vi "Capture.vi"(0 "Commands array":string[][](array[string])=[["Group20.825", "Group20.671", "Group20.814", "Group30.121"], ["Group2-0.528", "Group2-1.243", "Group2-0.539", "Group30.121"], ["Group20.374", "Group21.573", "Group20.363", "Group30.121"], ["Group2-0.242", "Group2-1.815", "Group2-0.253", "Group30.121"], ["Group20.165", "Group21.991", "Group20.154", "Group30.121"], ["Group2-0.077", "Group2-2.145", "Group2-0.088", "Group30.121"], ["Group20.044", "Group22.233", "Group20.033", "Group30.121"], ["Group2-2.310", "WT10", "WT10", "Group30.121"], ["Group22.310", "WT10", "WT10", "Group30.121"], ["Group2-2.310", "WT10", "WT10", "Group30.121"], ["Group22.310", "WT10", "WT10", "Group30.121"], ["Group2-2.310", "WT10", "WT10", "Group30.121"], ["Group22.310", "WT10", "WT10", "Group30.121"], ["Group2-0.011", "Group2-2.277", "Group2-0.022", "Group30.121"], ["Group20.066", "Group22.189", "Group20.055", "Group30.121"], ["Group2-0.121", "Group2-2.057", "Group2-0.132", "Group30.121"], ["Group20.209", "Group21.903", "Group20.198", "Group30.121"], ["Group2-0.297", "Group2-1.705", "Group2-0.308", "Group30.121"], ["Group20.451", "Group21.419", "Group20.440", "Group30.121"], ["Group2-0.660", "Group2-0.979", "Group2-0.671", "Group30.121"]], 1 "XPS_Address":string="192.168.254.254", 2 "VISA resource name":refnum<visa-resource-name>, 3 "laser array index":i32, 4 "Process time":dbl format="%#_13g", 5 "Axis Speed":dbl=1.0 format="%#_13g", 6 "Laser on/off array":bool[][](array[boolean])=[[FALSE, TRUE, FALSE, FALSE], [FALSE, TRUE, FALSE, FALSE], [FALSE, TRUE, FALSE, FALSE], [FALSE, TRUE, FALSE, FALSE], [FALSE, TRUE, FALSE, FALSE], [FALSE, TRUE, FALSE, FALSE], [FALSE, TRUE, FALSE, FALSE], [TRUE, FALSE, FALSE, FALSE], [TRUE, FALSE, FALSE, FALSE], [TRUE, FALSE, FALSE, FALSE], [TRUE, FALSE, FALSE, FALSE], [TRUE, FALSE, FALSE, FALSE], [TRUE, FALSE, FALSE, FALSE], [FALSE, TRUE, FALSE, FALSE], [FALSE, TRUE, FALSE, FALSE], [FALSE, TRUE, FALSE, FALSE], [FALSE, TRUE, FALSE, FALSE], [FALSE, TRUE, FALSE, FALSE], [FALSE, TRUE, FALSE, FALSE], [FALSE, TRUE, FALSE, FALSE]], 7 "stop":bool, 8 "delay before read (ms)":u32=500, 11 "Axis Initial Parameters":T1={"Velocity (units/seconds)"=1.0, "Acceleration (units/seconds²)"=20.0, "Minimum Jerk Time (seconds)"=0.005, "Maximum Jerk Time (seconds)"=0.009} {"Maximum Jerk Time (seconds)" format="%.6e"; "Minimum Jerk Time (seconds)" format="%.6e"; "Acceleration (units/seconds²)" format="%.6e"; "Velocity (units/seconds)" format="%.6e"}, 13 "ROI Area \n(mm2)":dbl=4.035870075999999, 14 "Axis 2":string="Group3", 15 "Axis 1":string="Group2", 17 "OPO on?":bool, 19 "Acceleration (units/seconds²)":dbl=20.0) -> (10 "Elapsed time":dbl, 16 "XPS error out":errorcluster, 18 "Error out":errorcluster)   [LabVIEW 2016]
uses:
  case selector.ctl
panel:
  out "Capture Log":string
  out "Axis 1 position":dbl format="%.10f"
  out "Axis 2 position":dbl format="%.10f"
  out "Initial time":timestamp
  in  "Active Positioner":string
  out "Current Line":i32
  out "1D Laser Array":bool[](array[boolean])=[FALSE, TRUE, FALSE, FALSE, FALSE, TRUE, FALSE, FALSE, FALSE, TRUE, FALSE, FALSE, FALSE, TRUE, FALSE, FALSE, FALSE, TRUE, FALSE, FALSE, FALSE, TRUE, FALSE, FALSE, FALSE, TRUE, FALSE, FALSE, TRUE, FALSE, FALSE, FALSE, TRUE, FALSE, FALSE, FALSE, TRUE, FALSE, FALSE, FALSE, TRUE, FALSE, FALSE, FALSE, TRUE, FALSE, FALSE, FALSE, TRUE, FALSE, FALSE, FALSE, FALSE, TRUE, FALSE, FALSE, FALSE, TRUE, FALSE, FALSE, FALSE, TRUE, FALSE, FALSE, FALSE, TRUE, FALSE, FALSE, FALSE, TRUE, FALSE, FALSE, FALSE, TRUE, FALSE, FALSE, FALSE, TRUE, FALSE, FALSE]
  out "1D command array":string[](array[string])=["Group20.825", "Group20.671", "Group20.814", "Group30.121", "Group2-0.528", "Group2-1.243", "Group2-0.539", "Group30.121", "Group20.374", "Group21.573", "Group20.363", "Group30.121", "Group2-0.242", "Group2-1.815", "Group2-0.253", "Group30.121", "Group20.165", "Group21.991", "Group20.154", "Group30.121", "Group2-0.077", "Group2-2.145", "Group2-0.088", "Group30.121", "Group20.044", "Group22.233", "Group20.033", "Group30.121", "Group2-2.310", "WT10", "WT10", "Group30.121", "Group22.310", "WT10", "WT10", "Group30.121", "Group2-2.310", "WT10", "WT10", "Group30.121", "Group22.310", "WT10", "WT10", "Group30.121", "Group2-2.310", "WT10", "WT10", "Group30.121", "Group22.310", "WT10", "WT10", "Group30.121", "Group2-0.011", "Group2-2.277", "Group2-0.022", "Group30.121", "Group20.066", "Group22.189", "Group20.055", "Group30.121", "Group2-0.121", "Group2-2.057", "Group2-0.132", "Group30.121", "Group20.209", "Group21.903", "Group20.198", "Group30.121", "Group2-0.297", "Group2-1.705", "Group2-0.308", "Group30.121", "Group20.451", "Group21.419", "Group20.440", "Group30.121", "Group2-0.660", "Group2-0.979", "Group2-0.671", "Group30.121"]
  out "Current Command":string
  out "Current laser element":bool
  out "Total lines":i32=80
  in  "Active Axis":string
  out "Laser on/off":bool
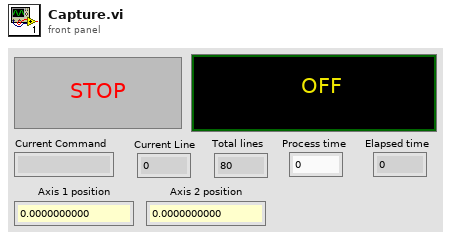
[diagram p1: front panel]
types:
  T1 = cluster{"Velocity (units/seconds)":dbl, "Acceleration (units/seconds²)":dbl, "Minimum Jerk Time (seconds)":dbl, "Maximum Jerk Time (seconds)":dbl}
  T2 = typedef "case selector.ctl" = enum16{"Initialize", "Element selection", "Laser", "Velocities", "Command", "Wait", "Exit"}
  T3 = enum16{"open", "replace", "create", "open or create", "replace or create", "replace or create with confirmation"}
  T4 = cluster{"connection TCP":refnum<k5>, "LogTo File":bool, "Log File refnum":refnum<file>, "no error if error log":bool}
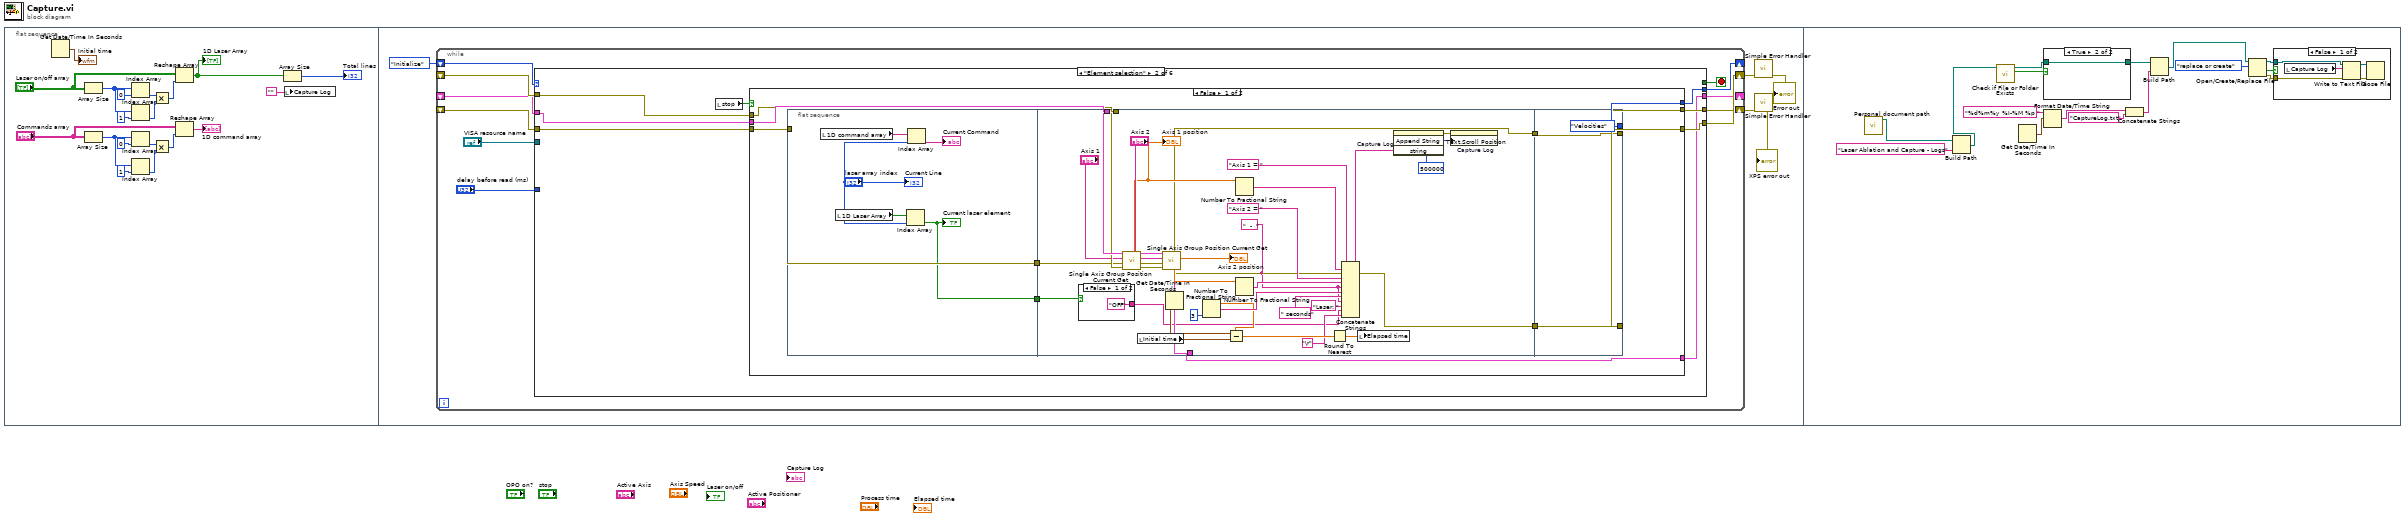
[diagram p0: block diagram]
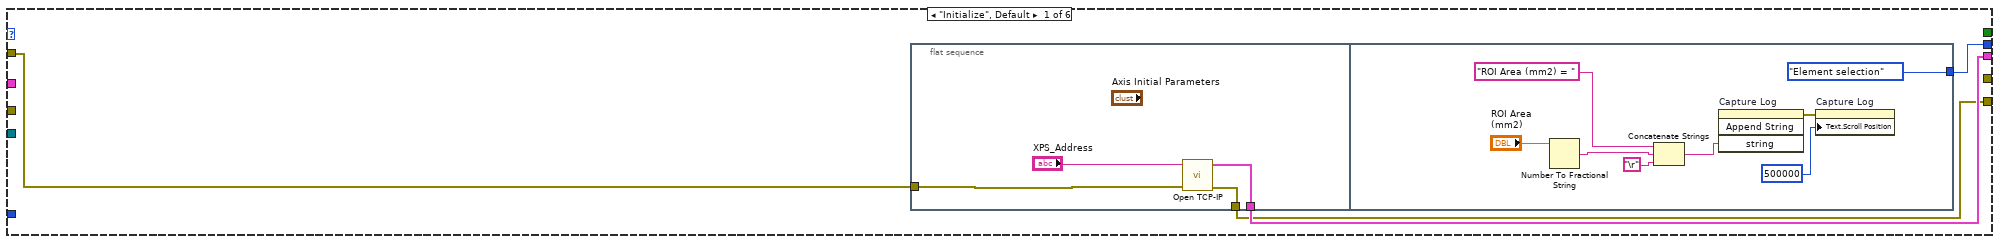
[diagram p2: hidden frame]
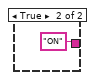
[diagram p3: hidden frame]
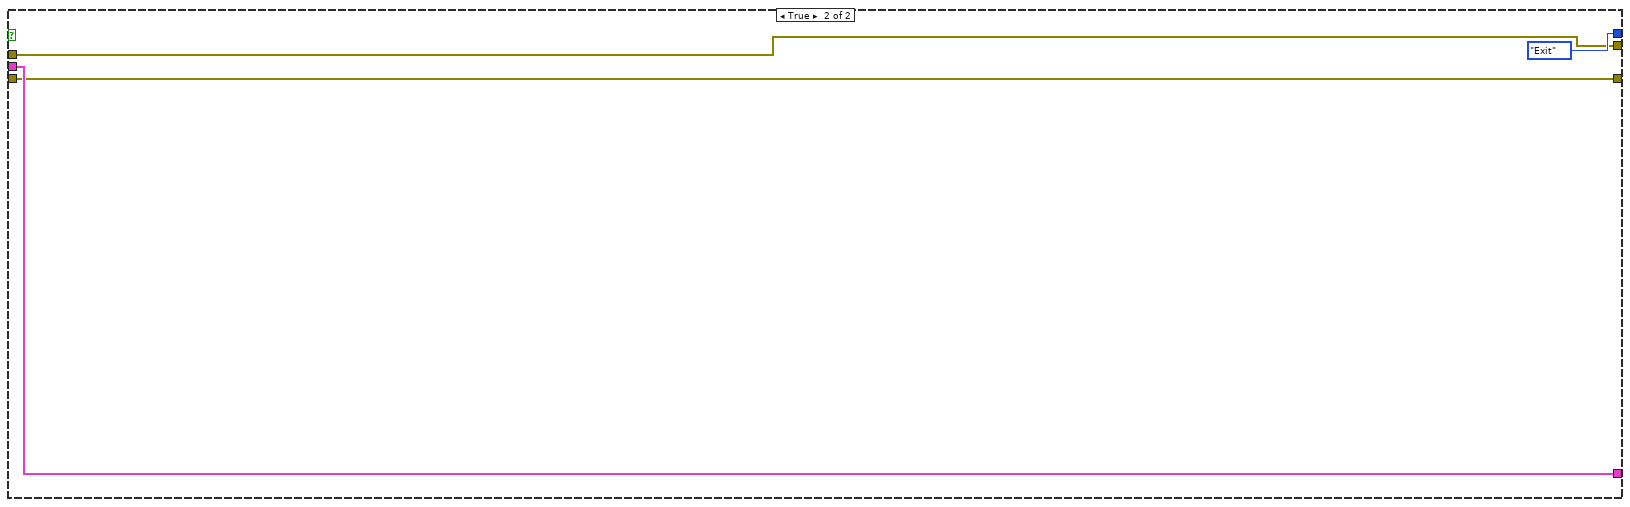
[diagram p4: hidden frame]
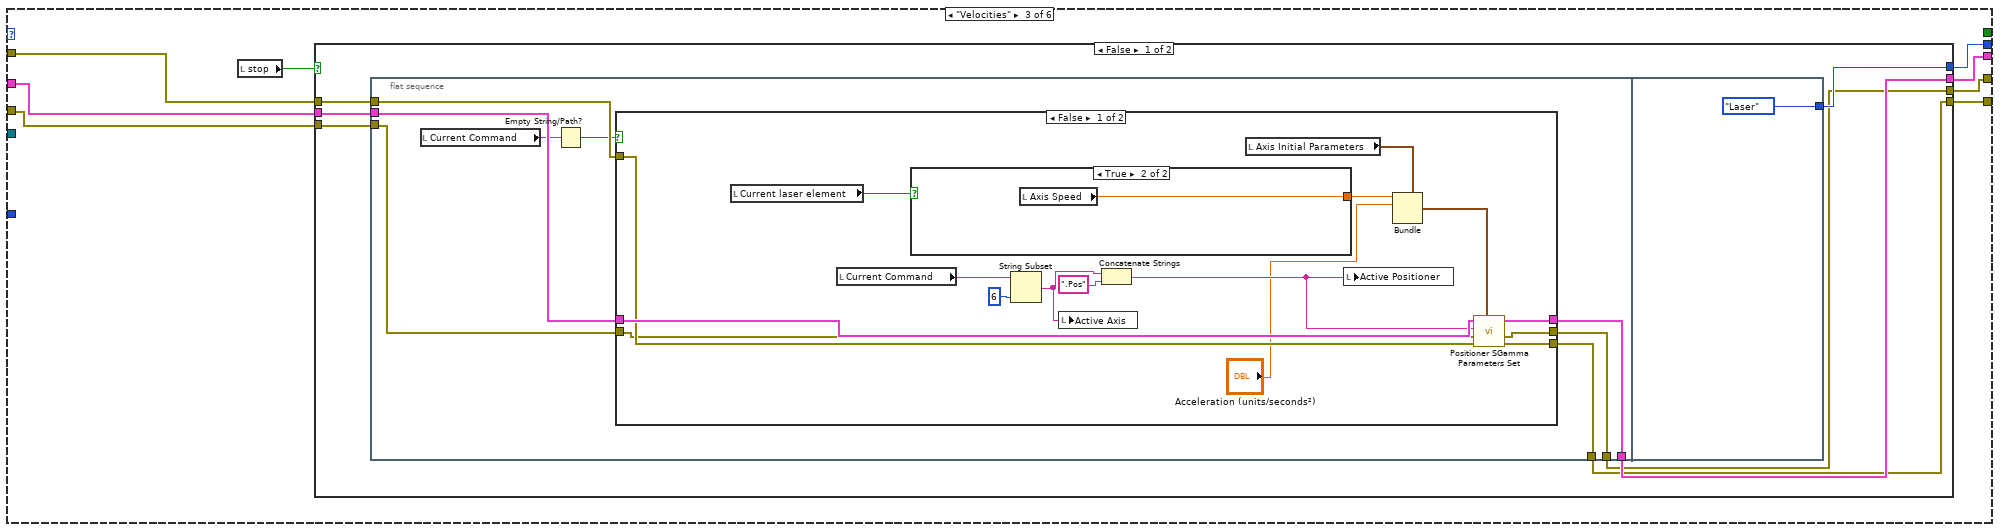
[diagram p5: hidden frame]
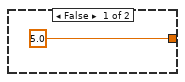
[diagram p6: hidden frame]
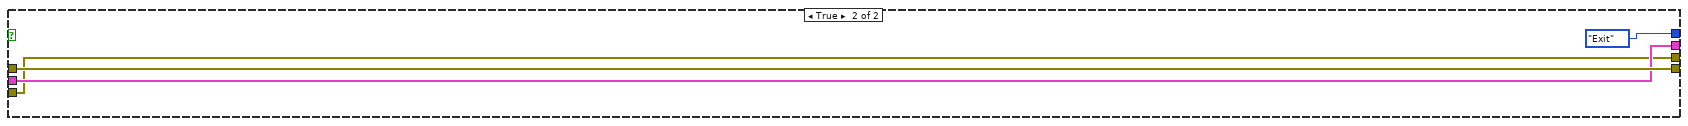
[diagram p8: hidden frame]
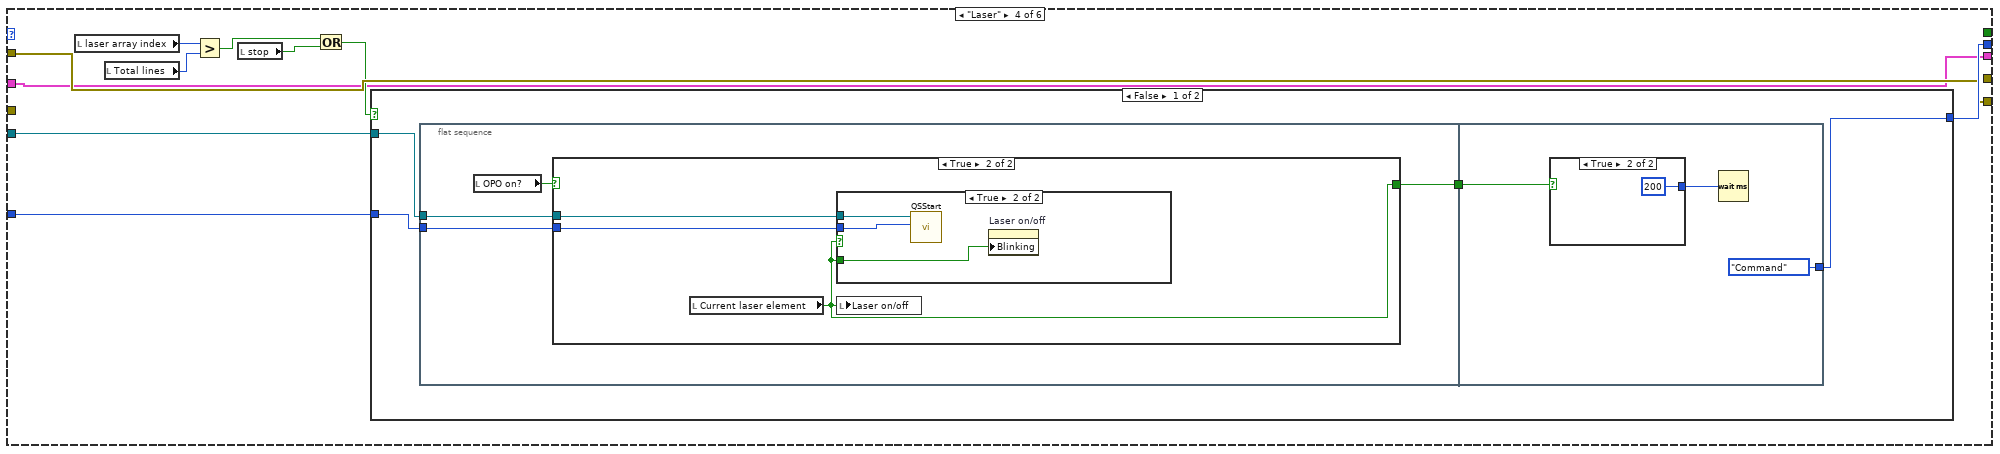
[diagram p9: hidden frame]
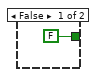
[diagram p10: hidden frame]
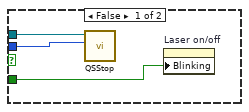
[diagram p11: hidden frame]
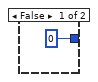
[diagram p12: hidden frame]
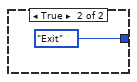
[diagram p13: hidden frame]
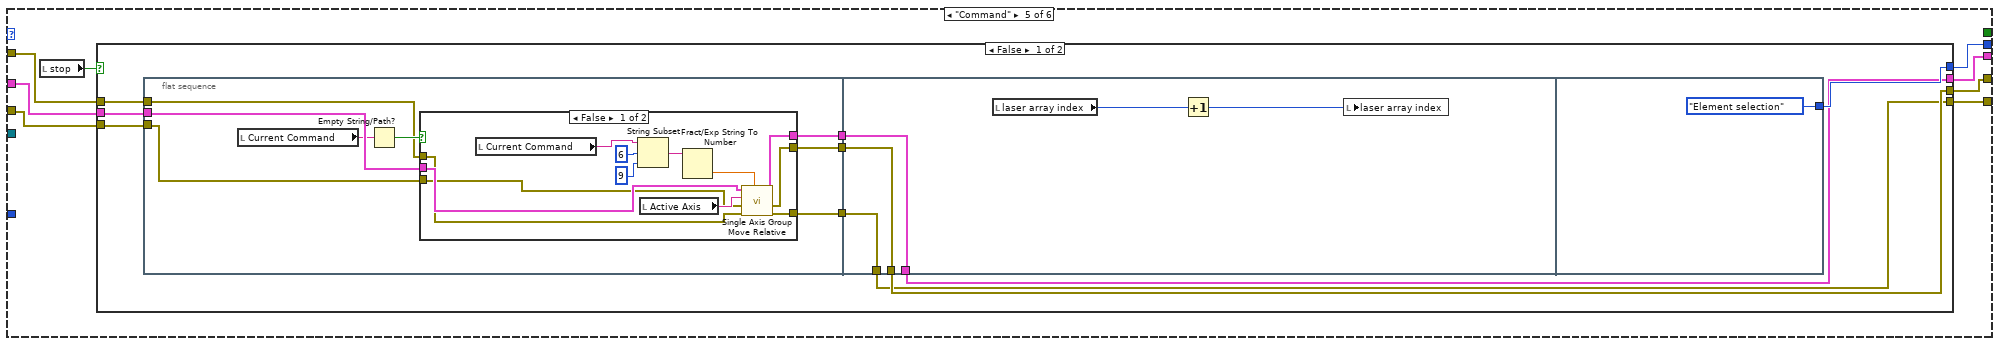
[diagram p14: hidden frame]
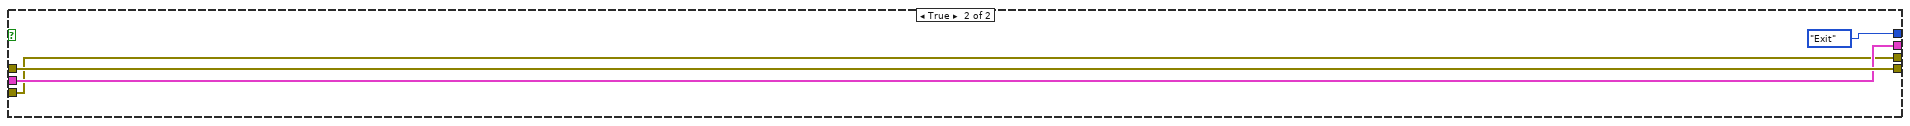
[diagram p16: hidden frame]
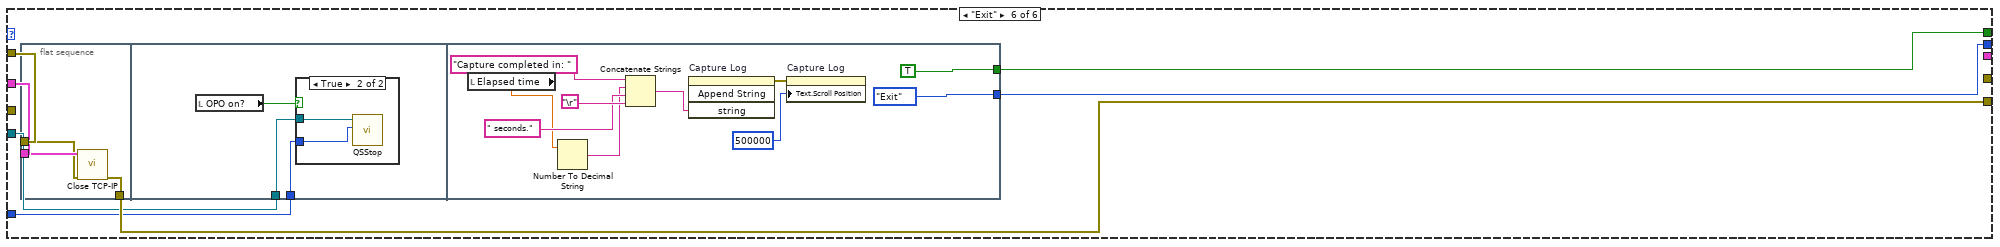
[diagram p17: hidden frame]
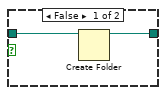
[diagram p19: hidden frame]
diagram:
  n1 = flat-sequence {
    frame #0 {
      n2 = Get Date/Time In Seconds() -> (seconds since 1Jan1904=→"Initial time":timestamp)
      n3 = Array Size(array="Commands array") -> (size(s)=w3:i32[])
      n4 = Array Size(array="Laser on/off array") -> (size(s)=w11:i32[])
      n5 = Index Array(array=w11, index=0) -> (element=w14:i32)
      n6 = Index Array(array=w11, index=1) -> (element=w15:i32)
      n7 = Index Array(array=w3, index=0) -> (element=w6:i32)
      n8 = Index Array(array=w3, index=1) -> (element=w7:i32)
      n9 = Multiply(x=w14, y=w15) -> (x*y=w16:i32)
      n10 = Multiply(x=w6, y=w7) -> (x*y=w8:i32)
      n11 = Reshape Array("Laser on/off array", w16) -> (w19:bool[])
      "1D Laser Array" <- w19
      n12 = Reshape Array("Commands array", w8) -> (→"1D command array":string[])
      n13 = Array Size(array=w19) -> (size(s)=→"Total lines":i32)
      n14 = local write "Capture Log"("") -> ()
    }
    frame #1 {
      n15 = while {
        shift-right: [w32] -> _
        shift-left: case_selector."Initialize" -> [w33]
        shift-right: [w30] -> w20
        shift-left: _ -> [w31]
        shift-right: [w29] -> _
        shift-left: _ -> [w28]
        shift-right: [w27] -> w21
        shift-left: _ -> [w26]
        stop <- w25 stop-if-true
        n16 = case shown="\"Element selection\"" w33 {
          tunnel: [w37 w57 w123 w174 w206 w253] -> w32
          tunnel: w31 -> [w36 w54 w121 w173 w204 w254]
          tunnel: [w34 w51 w120 w173 w203 w252] -> w30
          tunnel: [w35 w50 w118 w167 w201 _] -> w29
          tunnel: w28 -> [_ w55 w119 w167 w202 w251]
          tunnel: [_ w52 w117 _ w199 _] -> w27
          tunnel: w26 -> [_ w53 w116 _ w200 _]
          tunnel: [_ _ _ _ _ w250] -> w25
          tunnel: "VISA resource name" -> [_ _ _ w166 _ w248]
          tunnel: "delay before read (ms)" -> [_ _ _ w165 _ w249]
          frame "Initialize", Default {
            n17 = flat-sequence {
              tunnel: w36 -> [w40]
              tunnel: [w39] -> w35
              tunnel: [w38] -> w34
              tunnel: [case_selector."Element selection"] -> w37
              frame #0 {
                n18 = call <userlib>:"Open TCP-IP.vi"("error in (no error)"=w40, "IP address"="XPS_Address") -> ("error out"=w38:errorcluster, "Connection ID"=w39:T4)  [unwired: 7 in, 1 out]
              }
              frame #1 {
                n19 = Number To Fractional String(number="ROI Area \n(mm2)") -> (F-format string=w45:string)  [unwired: 3 in]
                n20 = Concatenate Strings("ROI Area (mm2) = " ("string"), w45, "\r") -> (w43:string)
                n21 = invoke on="Capture Log" class="Str" method="Append String"("string"=w43) -> (error out=w47:errorcluster)  [unwired: 3 in, 3 out]
                n22 = property on="Capture Log" class="Str"(error in=w47, "Text.Scroll Position"=u32 500000) -> ()  [unwired: 1 in, 2 out]
              }
            }
          }
          frame "Element selection" {
            n23 = local read "stop"() -> (w56:bool)
            n24 = case shown="False" w56 {
              tunnel: [w67 case_selector."Exit"] -> w57
              tunnel: w55 -> [w68 w114]
              tunnel: w54 -> [w61 w113]
              tunnel: w53 -> [w60 w112]
              tunnel: [w62 w113] -> w52
              tunnel: [w64 w112] -> w51
              tunnel: [w66 w114] -> w50
              frame False {
                n25 = flat-sequence {
                  tunnel: w60 -> [w70]
                  tunnel: [w70] -> w59
                  tunnel: [w69] -> w58
                  tunnel: w68 -> [w99]
                  tunnel: w61 -> [w97]
                  tunnel: [w90] -> w66
                  tunnel: [w89] -> w65
                  tunnel: [w88] -> w63
                  tunnel: w59 -> [w87]
                  tunnel: w58 -> [w75]
                  tunnel: [case_selector."Velocities"] -> w67
                  tunnel: w65 -> [w110]
                  tunnel: [w110] -> w64
                  tunnel: w63 -> [w109]
                  tunnel: [w109] -> w62
                  frame #0 {
                    n26 = local read "1D command array"() -> (w73:string[])
                    n27 = local read "1D Laser Array"() -> (w72:bool[])
                    n28 = Index Array(array=w72, index="laser array index") -> (element=w69:bool)
                    "Current laser element" <- w69
                    n29 = Index Array(array=w73, index="laser array index") -> (element=→"Current Command":string)
                    "Current Line" <- "laser array index"
                  }
                  frame #1 {
                    w79 = "  -  " ("string")
                    n30 = case shown="False" w75 {
                      tunnel: ["OFF" "ON"] -> w76
                      frame False {
                      }
                      frame True {
                      }
                    }
                    n31 = call <userlib>:"Single Axis Group Position Current Get.vi"("error in (no error)"=w97, "XPS error in (no error)"=w87, "SingleAxis Group  Name (250 c max)"="Axis 1", "connection ID in"=w99) -> ("error out"=w91:errorcluster, "XPS error out"=w92:errorcluster, "Current Position (units)"=w96:dbl, "connection ID out"=w93:T4)  [unwired: 4 in]
                    "Axis 1 position" <- w96
                    n32 = local read "Initial time"() -> (w84:timestamp)
                    n33 = call <userlib>:"Single Axis Group Position Current Get.vi"("error in (no error)"=w91, "XPS error in (no error)"=w92, "SingleAxis Group  Name (250 c max)"="Axis 2", "connection ID in"=w93) -> ("error out"=w89:errorcluster, "XPS error out"=w88:errorcluster, "Current Position (units)"=w95:dbl, "connection ID out"=w90:T4)  [unwired: 4 in]
                    "Axis 2 position" <- w95
                    n34 = Get Date/Time In Seconds() -> (seconds since 1Jan1904=w85:timestamp)
                    n35 = Subtract(x=w85, y=w84) -> (x-y=w81:dbl)
                    n36 = Number To Fractional String(number=w81, precision (6)=i16 3) -> (F-format string=w83:string)  [unwired: 2 in]
                    n37 = Number To Fractional String(number=w96) -> (F-format string=w105:string)  [unwired: 3 in]
                    n38 = Number To Fractional String(number=w95) -> (F-format string=w104:string)  [unwired: 3 in]
                    n39 = Round To Nearest(number=w81) -> (nearest integer value=w86:dbl)
                    n40 = Concatenate Strings("Axis 1 = " ("string"), w105, w79, "Axis 2 = " ("string"), w104, w79, w83, " seconds" ("milliseconds"), w79, "Laser: " ("string"), w76, "\r") -> (w102:string)
                    n41 = local write "Elapsed time"(w86) -> ()
                    n42 = invoke on="Capture Log" class="Str" method="Append String"("string"=w102) -> (error out=w101:errorcluster)  [unwired: 3 in, 3 out]
                    n43 = property on="Capture Log" class="Str"(error in=w101, "Text.Scroll Position"=u32 500000) -> ()  [unwired: 1 in, 2 out]
                  }
                  frame #2 {
                  }
                }
              }
              frame True {
              }
            }
          }
          frame "Velocities" {
            n44 = local read "stop"() -> (w122:bool)
            n45 = case shown="False" w122 {
              tunnel: [w130 case_selector."Exit"] -> w123
              tunnel: w121 -> [w129 w163]
              tunnel: [w126 w163] -> w120
              tunnel: w119 -> [w128 w162]
              tunnel: [w127 w162] -> w118
              tunnel: [w125 w161] -> w117
              tunnel: w116 -> [w124 w161]
              frame False {
                n46 = flat-sequence {
                  tunnel: w129 -> [w136]
                  tunnel: w128 -> [w138]
                  tunnel: [w137] -> w127
                  tunnel: [w135] -> w126
                  tunnel: [w134] -> w125
                  tunnel: w124 -> [w133]
                  tunnel: [case_selector."Laser"] -> w130
                  frame #0 {
                    n47 = local read "Current Command"() -> (w132:string)
                    n48 = Empty String/Path?(string/path=w132) -> (empty?=w131:bool)
                    n49 = case shown="False" w131 {
                      tunnel: w138 -> [w151 w157]
                      tunnel: [w150 w157] -> w137
                      tunnel: w136 -> [w149 w158]
                      tunnel: [w148 w158] -> w135
                      tunnel: [w143 w159] -> w134
                      tunnel: w133 -> [w142 w159]
                      frame False {
                        n50 = local read "Current laser element"() -> (w154:bool)
                        n51 = local read "Current Command"() -> (w152:string)
                        n52 = case shown="True" w154 {
                          tunnel: [5.0 w156] -> w147
                          frame False {
                          }
                          frame True {
                            n53 = local read "Axis Speed"() -> (w156:dbl)
                          }
                        }
                        n54 = String Subset(string=w152, length (rest)=6 ("length (rest)")) -> (substring=w141:string)  [unwired: 1 in]
                        n55 = local write "Active Axis"(w141) -> ()
                        n56 = Concatenate Strings(w141, ".Pos" ("string")) -> (w140:string)
                        n57 = local read "Axis Initial Parameters"() -> (w145:T1)
                        n58 = local write "Active Positioner"(w140) -> ()
                        n59 = Bundle(cluster=w145, "Velocity (units/seconds)"=w147, "Acceleration (units/seconds²)"="Acceleration (units/seconds²)") -> (w146:T1)  [unwired: 2 in]
                        n60 = call <userlib>:"Positioner SGamma Parameters Set.vi"("SGamma Parameters"=w146, "error in (no error)"=w149, "XPS error in (no error)"=w142, "Positioner Name (250 c max)"=w140, "connection ID in"=w151) -> ("error out"=w148:errorcluster, "XPS error out"=w143:errorcluster, "connection ID out"=w150:T4)  [unwired: 4 in]
                      }
                      frame True {
                      }
                    }
                  }
                  frame #1 {
                  }
                }
              }
              frame True {
              }
            }
          }
          frame "Laser" {
            n61 = local read "laser array index"() -> (w171:i32)
            n62 = local read "Total lines"() -> (w172:i32)
            n63 = Greater?(x=w171, y=w172) -> (0:w169:bool)
            n64 = local read "stop"() -> (w170:bool)
            n65 = Or(x=w169, y=w170) -> (x .or. y?=w168:bool)
            n66 = case shown="False" w168 {
              tunnel: [w178 case_selector."Exit"] -> w174
              tunnel: w166 -> [w176 _]
              tunnel: w165 -> [w175 _]
              frame False {
                n67 = flat-sequence {
                  tunnel: [w181] -> w177
                  tunnel: w176 -> [w180]
                  tunnel: w175 -> [w179]
                  tunnel: [case_selector."Command"] -> w178
                  tunnel: w177 -> [w194]
                  frame #0 {
                    n68 = local read "OPO on?"() -> (w182:bool)
                    n69 = case shown="True" w182 {
                      tunnel: [FALSE ("Current laser element") w186] -> w181
                      tunnel: w180 -> [_ w185]
                      tunnel: w179 -> [_ w184]
                      frame False {
                      }
                      frame True {
                        n70 = local read "Current laser element"() -> (w186:bool)
                        n71 = case shown="True" w186 {
                          tunnel: w186 -> [w189 w192]
                          tunnel: w185 -> [w188 w191]
                          tunnel: w184 -> [w187 w190]
                          frame False {
                            n72 = call "QSStop.vi"("delay before read (ms)"=w187, "VISA resource name"=w188) -> ()  [unwired: 6 in, 4 out]
                            n73 = property on="Laser on/off" class="Bool (strict)"("Blinking"=w189) -> ()  [unwired: 2 in, 2 out]
                          }
                          frame True {
                            n74 = call "QSStart.vi"("delay before read (ms)"=w190, "VISA resource name"=w191) -> ()  [unwired: 6 in, 4 out]
                            n75 = property on="Laser on/off" class="Bool (strict)"("Blinking"=w192) -> ()  [unwired: 2 in, 2 out]
                          }
                        }
                        n76 = local write "Laser on/off"(w186) -> ()
                      }
                    }
                  }
                  frame #1 {
                    n77 = case shown="True" w194 {
                      tunnel: [u32 0 ("milliseconds to wait") u32 200 ("milliseconds to wait")] -> w193
                      frame False {
                      }
                      frame True {
                      }
                    }
                    n78 = Wait (ms)(milliseconds to wait=w193) -> ()  [unwired: 1 out]
                  }
                }
              }
              frame True {
              }
            }
          }
          frame "Command" {
            n79 = local read "stop"() -> (w205:bool)
            n80 = case shown="False" w205 {
              tunnel: [w210 case_selector."Exit"] -> w206
              tunnel: w204 -> [w214 w246]
              tunnel: [w208 w246] -> w203
              tunnel: w202 -> [w216 w245]
              tunnel: [w207 w245] -> w201
              tunnel: w200 -> [w213 w244]
              tunnel: [w209 w244] -> w199
              frame False {
                n81 = flat-sequence {
                  tunnel: w216 -> [w224]
                  tunnel: [w223] -> w215
                  tunnel: w214 -> [w220]
                  tunnel: w213 -> [w219]
                  tunnel: [w218] -> w212
                  tunnel: [w217] -> w211
                  tunnel: w215 -> [w238]
                  tunnel: w212 -> [w240]
                  tunnel: w211 -> [w239]
                  tunnel: [w240] -> w209
                  tunnel: [w239] -> w208
                  tunnel: [w238] -> w207
                  tunnel: [case_selector."Element selection"] -> w210
                  frame #0 {
                    n82 = local read "Current Command"() -> (w221:string)
                    n83 = Empty String/Path?(string/path=w221) -> (empty?=w222:bool)
                    n84 = case shown="False" w222 {
                      tunnel: w224 -> [w236 w237]
                      tunnel: [w229 w237] -> w223
                      tunnel: w220 -> [w228 _]
                      tunnel: w219 -> [w227 _]
                      tunnel: [w226 _] -> w218
                      tunnel: [w225 _] -> w217
                      frame False {
                        n85 = local read "Current Command"() -> (w235:string)
                        n86 = String Subset(string=w235, offset (0)=6, length (rest)=9 ("length (rest)")) -> (substring=w232:string)
                        n87 = local read "Active Axis"() -> (w230:string)
                        n88 = Fract/Exp String To Number(string=w232) -> (number=w231:dbl)  [unwired: 3 in, 1 out]
                        n89 = call <userlib>:"Single Axis Group Move Relative.vi"("Target Displacement (units)"=w231, "error in (no error)"=w228, "XPS error in (no error)"=w227, "SingleAxis Group  Name (250 c max)"=w230, "connection ID in"=w236) -> ("error out"=w225:errorcluster, "XPS error out"=w226:errorcluster, "connection ID out"=w229:T4)  [unwired: 4 in]
                      }
                      frame True {
                      }
                    }
                  }
                  frame #1 {
                    n90 = local read "laser array index"() -> (w242:i32)
                    n91 = Increment(x=w242) -> (x+1=w241:i32)
                    n92 = local write "laser array index"(w241) -> ()
                  }
                  frame #2 {
                  }
                }
              }
              frame True {
              }
            }
          }
          frame "Exit" {
            n93 = flat-sequence {
              tunnel: w254 -> [w256]
              tunnel: [w255] -> w252
              tunnel: w251 -> [w257]
              tunnel: w249 -> [w259]
              tunnel: w248 -> [w258]
              tunnel: [case_selector."Exit"] -> w253
              tunnel: [TRUE] -> w250
              frame #0 {
                n94 = call <userlib>:"Close TCP-IP.vi"("error in (no error)"=w256, "connection ID in"=w257) -> ("Error out"=w255:errorcluster)  [unwired: 9 in]
              }
              frame #1 {
                n95 = local read "OPO on?"() -> (w260:bool)
                n96 = case shown="True" w260 {
                  tunnel: w259 -> [_ w262]
                  tunnel: w258 -> [_ w261]
                  frame False {
                  }
                  frame True {
                    n97 = call "QSStop.vi"("delay before read (ms)"=w262, "VISA resource name"=w261) -> ()  [unwired: 6 in, 4 out]
                  }
                }
              }
              frame #2 {
                n98 = local read "Elapsed time"() -> (w264:dbl)
                n99 = Number To Decimal String(number=w264) -> (decimal integer string=w263:string)  [unwired: 1 in]
                n100 = Concatenate Strings("Capture completed in: " ("string"), w263, " seconds." ("string"), "\r") -> (w265:string)
                n101 = invoke on="Capture Log" class="Str" method="Append String"("string"=w265) -> (error out=w270:errorcluster)  [unwired: 3 in, 3 out]
                n102 = property on="Capture Log" class="Str"(error in=w270, "Text.Scroll Position"=u32 500000) -> ()  [unwired: 1 in, 2 out]
              }
            }
          }
        }
      }
      "XPS error out" <- w21
      "Error out" <- w20
      n103 = call <vilib>:"Simple Error Handler.vi"("error in (no error)"=w20) -> ()  [unwired: 4 in, 5 out]
      n104 = call <vilib>:"Simple Error Handler.vi"("error in (no error)"=w21) -> ()  [unwired: 4 in, 5 out]
    }
    frame #2 {
      n105 = call "Personal document path.vi"() -> ("My Documents"=w274:path)  [unwired: 10 in, 1 out]
      n106 = Build Path(base path=w274, name or relative path="Laser Ablation and Capture - Logs") -> (appended path=w273:path)
      n107 = call <vilib>:"Check if File or Folder Exists.vi"("path"=w273) -> ("file or folder exists?"=w283:bool, "dup path"=w282:path)  [unwired: 8 in, 1 out]
      n108 = Get Date/Time In Seconds() -> (seconds since 1Jan1904=w285:timestamp)
      n109 = case shown="True" w283 {
        tunnel: w282 -> [w290 w291]
        tunnel: [w289 w291] -> w279
        frame False {
          n110 = Create Folder(path (use dialog)=w290) -> (created path=w289:path)  [unwired: 2 in, 2 out]
        }
        frame True {
        }
      }
      n111 = Format Date/Time String(time format string (%c)="%d%m%y %I-%M %p ", seconds (now)=w285) -> (date/time string=w287:string)  [unwired: 1 in]
      n112 = Concatenate Strings(w287, "CaptureLog.txt") -> (w280:string)
      n113 = Build Path(base path=w279, name or relative path=w280) -> (appended path=w281:path)
      n114 = Open/Create/Replace File(file path (use dialog)=w281, operation (0:open)=T3."replace or create") -> (refnum out=w278:refnum<file>, cancelled=w276:bool, error out=w277:errorcluster)  [unwired: 4 in]
      n115 = case shown="False" w276 {
        tunnel: w278 -> [w296 _]
        tunnel: w277 -> [w294 _]
        frame False {
          n116 = local read "Capture Log"() -> (w295:string)
          n117 = Write to Text File(file (use dialog)=w296, text=w295, error in=w294) -> (refnum out=w293:refnum<file>, error out=w292:errorcluster)  [unwired: 2 out]
          n118 = Close File(refnum=w293, error in=w292) -> ()  [unwired: 2 out]
        }
        frame True {
        }
      }
    }
  }
